vi "Host - Scan next ECAT Slave Level.vi"(8 "Fehler (Eingang, kein Fehler)":errorcluster, 11 "Array (Eingang)":refnum<k21>[](array[refnum])) -> (0 "Fehler (Ausgang)":errorcluster, 3 "Array (Ausgang)":refnum<k21>[](array[refnum]))   [LabVIEW 2016, in "Scan Engine Custom Device.lvlib"]
uses:
  Scan Engine Custom Device.lvlib
  <resource>/objmgr/IndComECAT.rc
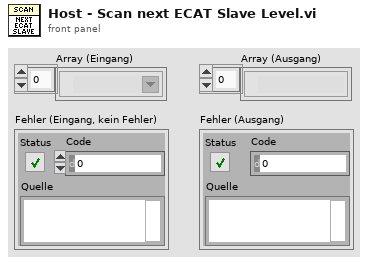
[diagram p1: front panel]
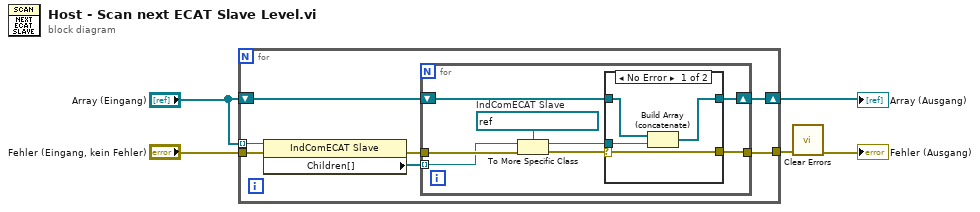
[diagram p0: block diagram]
diagram:
  n1 = for {
    shift-right: [w12] -> w5
    shift-left: "Array (Eingang)" -> [w11]
    tunnel: [w10] -> w4
    tunnel: "Array (Eingang)" -> [w8] mode=indexing
    tunnel: "Fehler (Eingang, kein Fehler)" -> [w9]
    n2 = property class="IndComECAT Slave"(reference=w8, error in=w9) -> (error out=w7:errorcluster, "Children[]"=w6:refnum<k21>[])  [unwired: 1 out]
    n3 = for {
      shift-right: [w19] -> w12
      shift-left: w11 -> [w18]
      tunnel: w6 -> [w13] mode=indexing
      tunnel: w7 -> [w14]
      tunnel: [w17] -> w10
      w20 = refnum<k21> refnum  # IndComECAT Slave
      n4 = To More Specific Class(target class=w20, reference=w13, error in=w14) -> (specific class reference=w15:refnum<k21>, error out=w16:errorcluster)
      n5 = case shown="No Error" w16 {
        selector: w16 -> [w21 w25]
        tunnel: w15 -> [w24 _]
        tunnel: [w23 w26] -> w19
        tunnel: w18 -> [w22 w26]
        tunnel: [w21 w25] -> w17
        frame No Error {
          n6 = Build Array (concatenate)(w22, w24) -> (w23:refnum<k21>[])
        }
        frame Error {
        }
      }
    }
  }
  "Array (Ausgang)" <- w5
  n7 = call <vilib>:"Clear Errors.vi"("error in (no error)"=w4) -> ("error out"=→"Fehler (Ausgang)":errorcluster)  [unwired: 5 in, 1 out]
